vi "Set Select App Event.vi"(8 "error in (no error)":errorcluster, 10 "Select App":refnum<user-event>, 11 "AppListPanel in":refnum<class "AppListPanel.lvclass">) -> (0 "error out":errorcluster, 3 "AppListPanel out":refnum<class "AppListPanel.lvclass">)   [LabVIEW 2020, in "PicoG-App.lvlib" / "AppListPanel.lvclass"]
uses:
  AppListPanel.lvclass
  ViaApp/ViaApp.lvclass
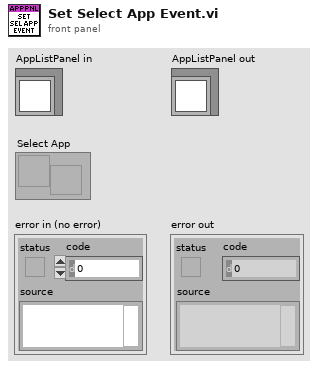
[diagram p1: front panel]
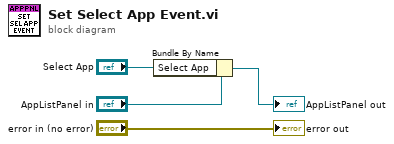
[diagram p0: block diagram]
diagram:
  n1 = Bundle By Name(cluster="AppListPanel in", "Select App"="Select App") -> (→"AppListPanel out":refnum<class "AppListPanel.lvclass">)
  "error out" <- "error in (no error)"
